vi "SPECTRUM Set Settings_AS2.vi"(2 "error in (no error)":errorcluster, 3 "Cluster":T1 {"verticalUnit" items=["SpectrumVerticalUnit_dBm", "SpectrumVerticalUnit_Watt", "SpectrumVerticalUnit_Volt", "SpectrumVerticalUnit_Amp", "SpectrumVerticalUnit_dBmV"]; "window" items=["SpectrumWindow_Kaiser", "SpectrumWindow_Mil6dB", "SpectrumWindow_BlackmanHarris", "SpectrumWindow_Rectangle", "SpectrumWindow_FlatTop", "SpectrumWindow_Hann"]; "traceLength" items=["801"=801, "2401"=2401, "4001"=4001, "8001"=8001, "10401"=10401, "16001"=16001, "32001"=32001, "64001"=64001]}) -> (0 "error out":errorcluster, 1 "function return":u32(ring))   [LabVIEW 2016]
doc: "RSA_API_DLL ReturnStatus SPECTRUM_SetSettings(Spectrum_Settings settings);"
uses:
  <userlib>/RSA_API/RSA_API.lvlib
  Tektronix/RSA_API/lib/x86/RSA_API.dll
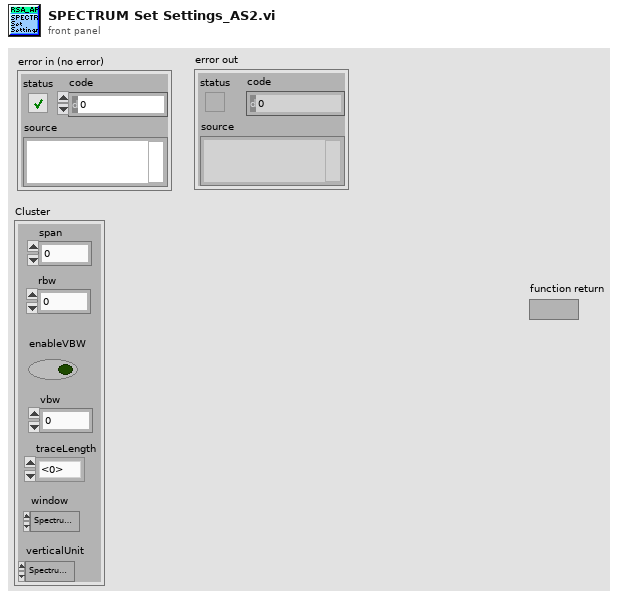
[diagram p1: front panel]
types:
  T1 = cluster{"span":dbl, "rbw":dbl, "enableVBW":bool, "vbw":dbl, "traceLength":u16, "window":u32, "verticalUnit":u32}
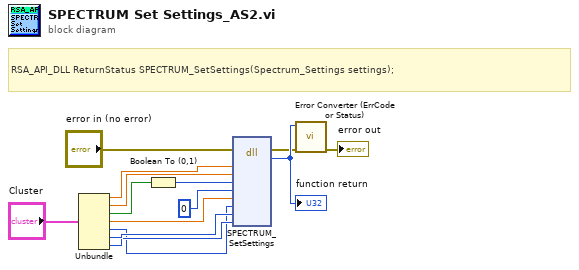
[diagram p0: block diagram]
diagram:
  # "RSA_API_DLL ReturnStatus SPECTRUM_SetSettings(Spectrum_Settings settings);"
  n1 = Unbundle("Cluster") -> ("span"=w9:dbl, "rbw"=w8:dbl, "enableVBW"=w7:bool, "vbw"=w6:dbl, "traceLength"=w1:u16, "window"=w5:u32, "verticalUnit"=w4:u32)
  n2 = Boolean To (0,1)(Boolean=w7) -> (0, 1=w13:i16)
  n3 = dll-call lib="C:/Tektronix/RSA_API/lib/x86/RSA_API.dll" fn="SPECTRUM_SetSettings"(error in="error in (no error)", "span"=w9, "rbw"=w8, "enableVBW"=w13, "@dummy control@"=i8 0, "vbw"=w6, "traceLength"=w1, "window"=w5, "verticalUnit"=w4) -> (error out=w12:errorcluster, "return type"=w14:u32)  [unwired: 10 in, 1 out]
  "function return" <- w14
  n4 = call <userlib>:"Error Converter (ErrCode or Status).vi"("error in (no error)"=w12, "error code"=w14) -> ("error out"=→"error out":errorcluster)  [unwired: 9 in]
